vi "ACQUIS_BASE_2015.vi"() -> ()   [LabVIEW 2014]
uses:
  <vilib>/DAQmx/read.llb/DAQmx Read (Analog Wfm 1Chan NSamp).vi
  <vilib>/DAQmx/create/channels.llb/DAQmx Create Channel (AI-Voltage-Basic).vi
  <vilib>/DAQmx/configure/timing.llb/DAQmx Timing (Sample Clock).vi
  <vilib>/DAQmx/miscellaneous.llb/DAQmx Fill In Error Info.vi
  <vilib>/Waveform/WDTFileIO.llb/Export Waveform To Spreadsheet File.vi
panel:
  in  "Boolean 2":bool
  out "Waveform Graph":waveform(dbl)(graph)
  in  "Campioni al s":dbl=10000.0
  in  "sample mode":i32(ring)=10178 items=["Finite Samples"=10178, "Continuous Samples"=10123, "Hardware Timed Single Point"=12522]
  in  "physical channels":tag="Dev1/ai0"
  in  "input terminal configuration":i32(ring)=10083 items=["Default"=-1, "RSE"=10083, "NRSE"=10078, "Differential"=10106, "Pseudodifferential"=12529]
  in  "Fondo Scala":dbl(ring)=10.0 items=["10"=10.0, "5"=5.0, "0.5"=0.5, "0.05"=0.05]
  in  "Durata (s)":dbl=0.1
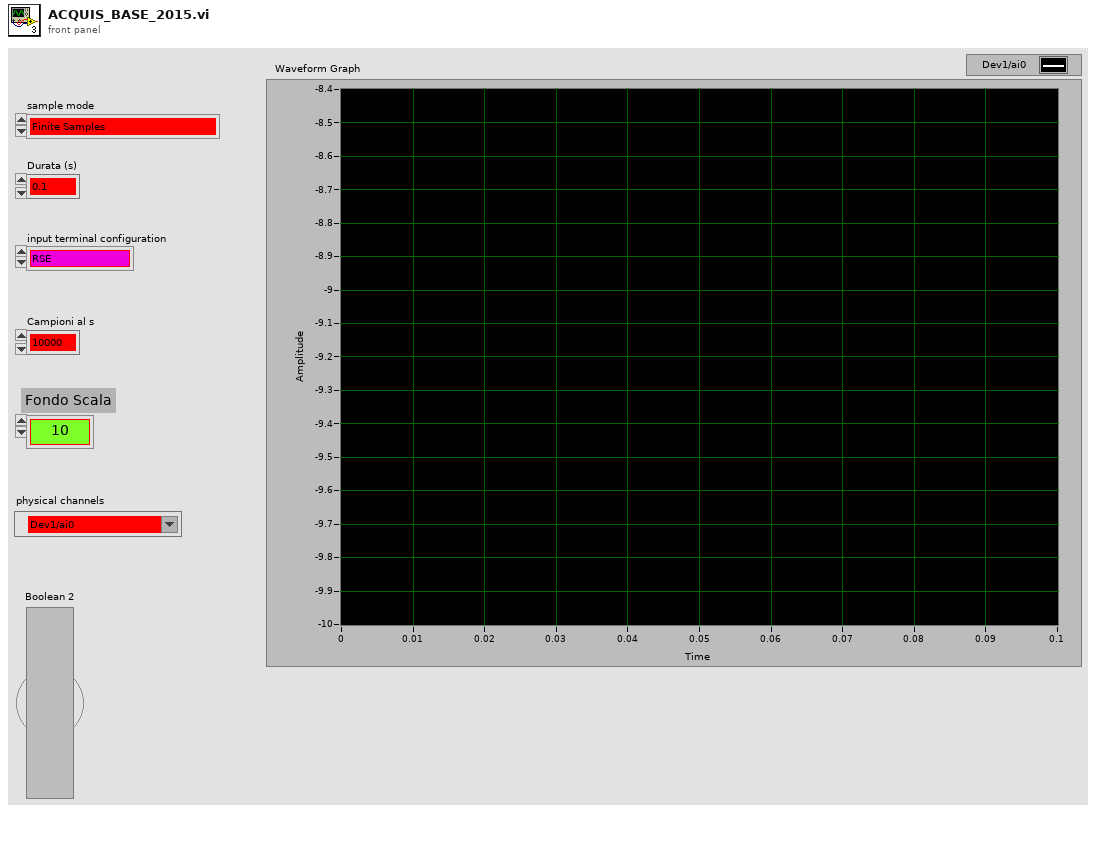
[diagram p1: front panel]
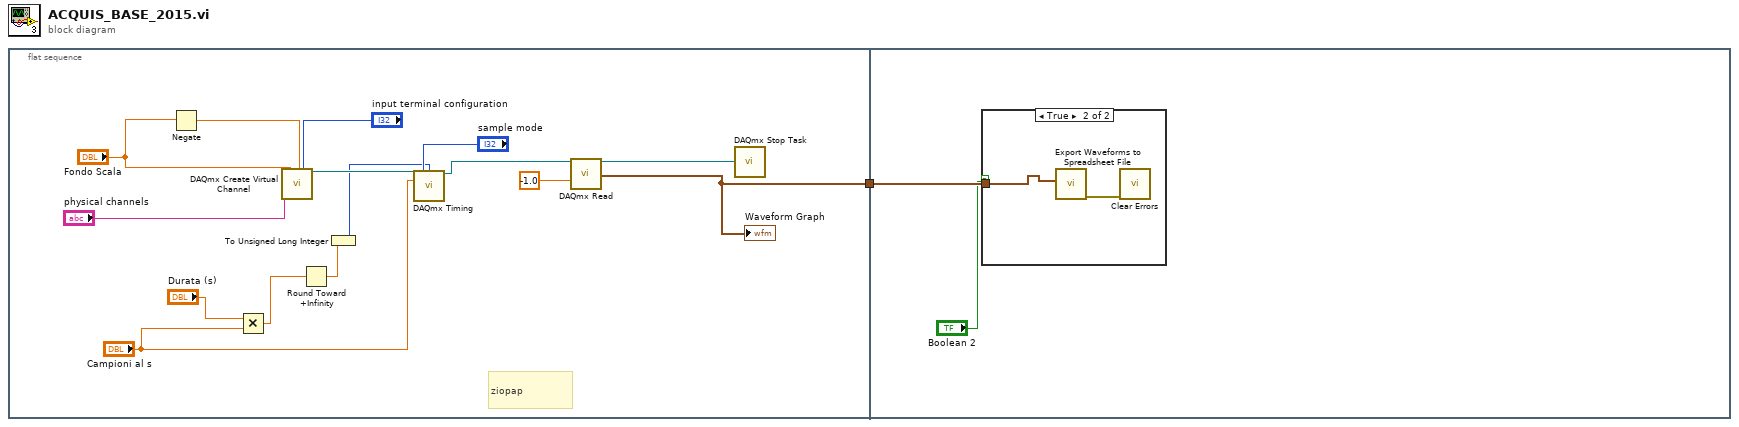
[diagram p0: block diagram]
diagram:
  n1 = flat-sequence {
    tunnel: [w2] -> w1
    tunnel: w1 -> [w18]
    frame #0 {
      # "ziopap"
      n2 = Negate(x="Fondo Scala") -> (-x=w12:dbl)
      n3 = Multiply(x="Durata (s)", y="Campioni al s") -> (x*y=w6:dbl)
      n4 = call-poly <vilib>:"DAQmx Create Virtual Channel.vi"("maximum value"="Fondo Scala", "minimum value"=w12, "input terminal configuration"="input terminal configuration", "physical channels"="physical channels") -> ("task out"=w16:refnum<k21>)  [unwired: 10 in, 1 out]
      n5 = Round Toward +Infinity(x=w6) -> (ceil(x): smallest int >= x=w5:dbl)
      n6 = To Unsigned Long Integer(number=w5) -> (unsigned 32bit integer=w4:u32)
      n7 = call-poly <vilib>:"DAQmx Timing.vi"("task/channels in"=w16, "sample mode"="sample mode", "samples per channel"=w4, "rate"="Campioni al s") -> ("task out"=w15:refnum<k21>)  [unwired: 10 in, 1 out]
      n8 = call-poly <vilib>:"DAQmx Read.vi"("task/channels in"=w15, "timeout"=-1.0) -> ("task out"=w14:refnum<k21>, "data"=w2:waveform(dbl))  [unwired: 11 in, 1 out]
      "Waveform Graph" <- w2
      n9 = call <vilib>:"DAQmx Stop Task.vi"("task/channels in"=w14) -> ()  [unwired: 13 in, 2 out]
    }
    frame #1 {
      n10 = case shown="True" "Boolean 2" {
        tunnel: w18 -> [_ w20]
        frame False {
        }
        frame True {
          n11 = call-poly <vilib>:"Export Waveforms to Spreadsheet File.vi"("waveform"=w20) -> ("error out"=w19:errorcluster)  [unwired: 9 in, 1 out]
          n12 = call <vilib>:"Clear Errors.vi"("error in (no error)"=w19) -> ()  [unwired: 5 in, 2 out]
        }
      }
    }
  }
